vi "Read One Data Log.vi"(8 "error in (no error)":errorcluster, 11 "VISA resource name":refnum<visa-resource-name>) -> (0 "error out":errorcluster, 2 "Logged Data":dbl[][](array[numeric]), 3 "VISA resource name out":refnum<visa-resource-name>)   [LabVIEW 2013]
doc: "Reads the data from the internal meter of the Watts Up device. Outputs a 2D array of values, where each row is its own 1D array of the data points for each different measurement type (Watts,Volts,Amps,etc).\n\n<b>Note:</b> This VI may take several minutes to complete."
uses:
  <instrlib>/Watts Up Series/Watts Up Series.lvlib
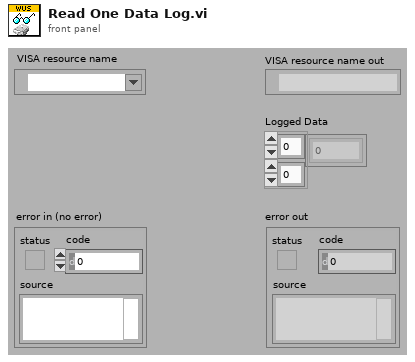
[diagram p1: front panel]
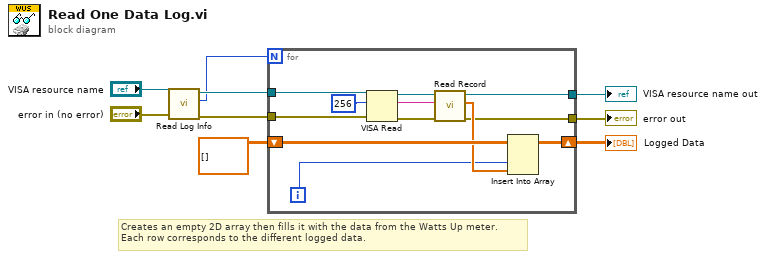
[diagram p0: block diagram]
diagram:
  # "Creates an empty 2D array then fills it with the data from the Watts Up meter.\nEach row corresponds to the different logged data."
  n1 = call <instrlib>:"Read Log Info.vi"("VISA resource name"="VISA resource name", "error in (no error)"="error in (no error)") -> ("VISA resource name out"=w9:refnum<visa-resource-name>, "Count"=w6:i32, "error out"=w8:errorcluster)  [unwired: 6 in]
  n2 = for {
    N: w6 -> [_]
    tunnel: w9 -> [w21]
    tunnel: w8 -> [w20]
    tunnel: [w15] -> w7
    shift-right: [w12] -> w4
    shift-left: dbl[][] [] -> [w14]
    tunnel: [w10] -> w3
    i -> [w11]
    n3 = VISA Read(VISA resource name=w21, byte count=u32 256, error in (no error)=w20) -> (VISA resource name out=w18:refnum<visa-resource-name>, read buffer=w17:string, error out=w16:errorcluster)  [unwired: 1 out]
    n4 = call <instrlib>:"Read Record.vi"("error in (no error)"=w16, "CSV String"=w17, "VISA resource name"=w18) -> ("error out"=w10:errorcluster, "Record"=w13:dbl[], "VISA resource name out"=w15:refnum<visa-resource-name>)  [unwired: 6 in]
    n5 = Insert Into Array(array=w14, index (col)=w11, new element=w13) -> (w12:dbl[][])  [unwired: 1 in]
  }
  "VISA resource name out" <- w7
  "error out" <- w3
  "Logged Data" <- w4
